vi "运维调试_采配水.vi"() -> ()   [LabVIEW 2016, in "PLC.lvlib"]
uses:
  PLC.lvlib
  <vilib>/Plasmionique/MB Master/MB_Master/MB_Master.lvclass
  <vilib>/Utility/miscctls.llb/LVPointTypeDef.ctl
  <vilib>/Plasmionique/MB Master/MB_Master_Serial/MB_Master_Serial.lvclass
  D:/Program Files (x86)/National Instruments/LabVIEW 2016/vi.lib/Plasmionique/MB Master/MB_Master/MB_Master.lvclass
  <vilib>/Utility/config.llb/Read Key (U32).vi
  <vilib>/Plasmionique/MB Master/MB Master.lvlib
  <vilib>/Utility/config.llb/NI_LVConfig.lvlib
panel:
  out "R21":i16
  in  "V7":bool
  out "R20":i16
  in  "M1-2":bool
  in  "潜水泵工作模式":u16(ring) items=["泵1单泵单管路", "泵2单泵单管路", "双泵双管路"]
  out "X10":bool caption="废液报警"
  out "X9":bool caption="自来水报警"
  out "X8":bool caption="泵2过载报警"
  out "X7":bool caption="泵1过载报警"
  out "X6":bool caption="断电检测"
  out "X5":bool caption="开门检测"
  out "X4":bool caption="烟雾检测"
  out "X3":bool caption="漏水检测"
  out "X2":bool caption="进样检测"
  out "X1":bool
  out "X0":bool caption="采样池液位开关"
  out "Y12":bool caption="多参通电"
  out "R109":i16 caption="配水时间"
  out "集成报警信息":string
  out "R108":i16 caption="自来水报警"
  out "R107":i16 caption="采水池液位报警设置"
  out "R106":i16 caption="进样超时设置"
  out "R105":i16 caption="二级清洗时间"
  out "R104":i16 caption="一级清洗时间"
  out "R103":i16 caption="外部管路清洗时间"
  out "R102":i16 caption="静置沉淀时间"
  out "R101":i16 caption="内部管路润洗时间"
  out "R100":i16 caption="外部管路润洗时间"
  out "R2":i16
  out "R1":i16
  out "多列列表框":i32(listbox)
  out "R19":i16
  in  "V6":bool
  out "R18":i16
  in  "V5":bool
  out "R17":i16
  in  "V4":bool
  out "R16":i16
  in  "V3":bool
  out "R15":i16
  in  "V2":bool
  out "R14":i16
  in  "M2":bool
  out "R13":i16
  in  "V1":bool
  out "R12":i16
  in  "M1-1":bool
  in  "返回":bool
  in  "参数设置":bool
  in  "单步启动":bool
  in  "启动":bool
  in  "停止":bool
  # "S"
  # "S"
  # "S"
  # "S"
  # "S"
  # "S"
  # "S"
  # "S"
  # "S"
  # "S"
  # "单步计时："
  # "s"
  # "流程计时："
  # "s"
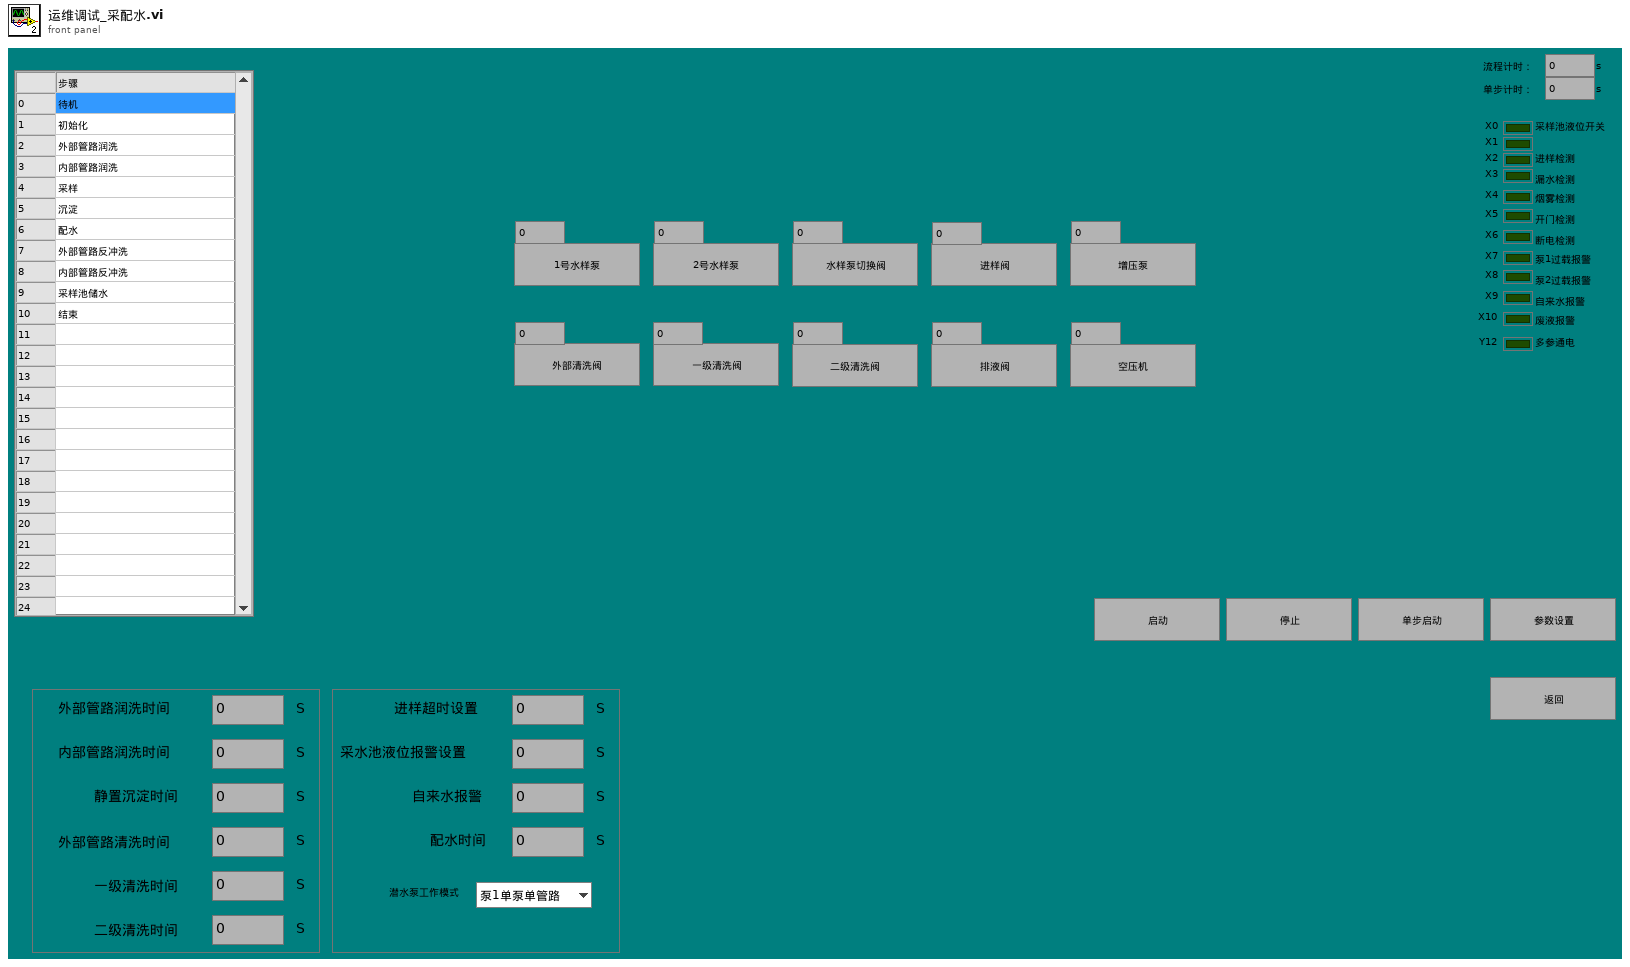
[diagram p1: front panel]
types:
  T1 = typedef "LVPointTypeDef.ctl" = cluster{"Horizontal":i16, "Vertical":i16}
  T2 = cluster{"时间标识":timestamp, "设备":string, "日志信息":string}
  T3 = cluster{"R0":i16, "R1":i16, "R2":i16, "R3":i16, "R4":i16, "R5":i16, "R6":i16, "R7":i16, "R8":i16, "R9":i16, "R10":i16, "R11":i16, "R12":i16, "R13":i16, "R14":i16, "R15":i16, "R16":i16, "R17":i16, "R18":i16, "R19":i16, "R20":i16, "R21":i16}
  T4 = cluster{"coil values[0]":bool, "coil values[1]":bool, "coil values[2]":bool, "coil values[3]":bool, "coil values[4]":bool, "coil values[5]":bool, "coil values[6]":bool, "coil values[7]":bool, "coil values[8]":bool, "coil values[9]":bool, "coil values[10]":bool, "coil values[11]":bool, "coil values[12]":bool, "coil values[13]":bool, "coil values[14]":bool, "coil values[15]":bool}
  T5 = cluster{"seconds since 1Jan1904":timestamp, "table输入":string, string, "table输入":string}
  T6 = cluster{"时间标识":timestamp, "设备":string, "日志信息":string, "流程参数":string}
  T7 = cluster{"命令":string, cluster{"starting address":u16, "holding register value":u16}}
  T8 = cluster{"是否启用仪器":bool, "CODMn":cluster{"启动测量模式":cluster{"测量模式":enum16{"水样测量", "标样核查", "零点核查", "加标回收", "平行样", "校零", "校标"}}, "确定按钮":bool}, "采水模式":enum16{"使用采水泵", "不使用采水泵"}}
  T9 = enum16{"水样测量", "标样核查", "零点核查", "加标回收", "平行样", "校零", "校标"}
  T10 = cluster{"命令":string, "数据":cluster{"starting address":u16, "holding register value":u16}}
  T11 = cluster{"命令":string, "数据":cluster{"starting address":u16, "holding register values":u16[]}}
  T12 = cluster{"命令":string, "data":cluster{"starting address":u16, "coil values":bool[]}}
  T13 = enum32{"Bad", "Idle", "Run top level", "Running"}
  T14 = typedef "NI_LVConfig.lvlib/Config Data RefNum.ctl" = refnum<k1>
  T15 = cluster{"baud rate (bps)":u32, "stop bits":u16, "parity":u16, "flow control":u16, "timeout":u32, "retries":i32}
  T16 = cluster{"starting address":u16, "holding register values":u16[]}
  T17 = cluster{"starting address":u16, "holding register value":u16}
  T18 = cluster{"starting address":u16, "coil values":bool[]}
  T19 = cluster{"Registers[0]":u16, "Registers[1]":u16, "Registers[2]":u16, "Registers[3]":u16, "Registers[4]":u16, "Registers[5]":u16, "Registers[6]":u16, "Registers[7]":u16, "Registers[8]":u16, "Registers[9]":u16, "Registers[10]":u16, "Registers[11]":u16, "Registers[12]":u16, "Registers[13]":u16, "Registers[14]":u16, "Registers[15]":u16, "Registers[16]":u16, "Registers[17]":u16, "Registers[18]":u16, "Registers[19]":u16, "Registers[20]":u16, "Registers[21]":u16}
  T20 = cluster{"Registers[0]":u16, "Registers[1]":u16, "Registers[2]":u16, "Registers[3]":u16, "Registers[4]":u16, "Registers[5]":u16}
  T21 = cluster{"Coils[0]":bool, "Coils[1]":bool, "Coils[2]":bool, "Coils[3]":bool, "Coils[4]":bool, "Coils[5]":bool, "Coils[6]":bool, "Coils[7]":bool, "Coils[8]":bool, "Coils[9]":bool, "Coils[10]":bool, "Coils[11]":bool, "Coils[12]":bool, "Coils[13]":bool, "Coils[14]":bool, "Coils[15]":bool}
  T22 = cluster{"Registers[0]":u16, "Registers[1]":u16, "Registers[2]":u16, "Registers[3]":u16, "Registers[4]":u16, "Registers[5]":u16, "Registers[6]":u16, "Registers[7]":u16, "Registers[8]":u16, "Registers[9]":u16, "Registers[10]":u16, "Registers[11]":u16, "Registers[12]":u16, "Registers[13]":u16, "Registers[14]":u16, "Registers[15]":u16, "Registers[16]":u16, "Registers[17]":u16, "Registers[18]":u16, "Registers[19]":u16}
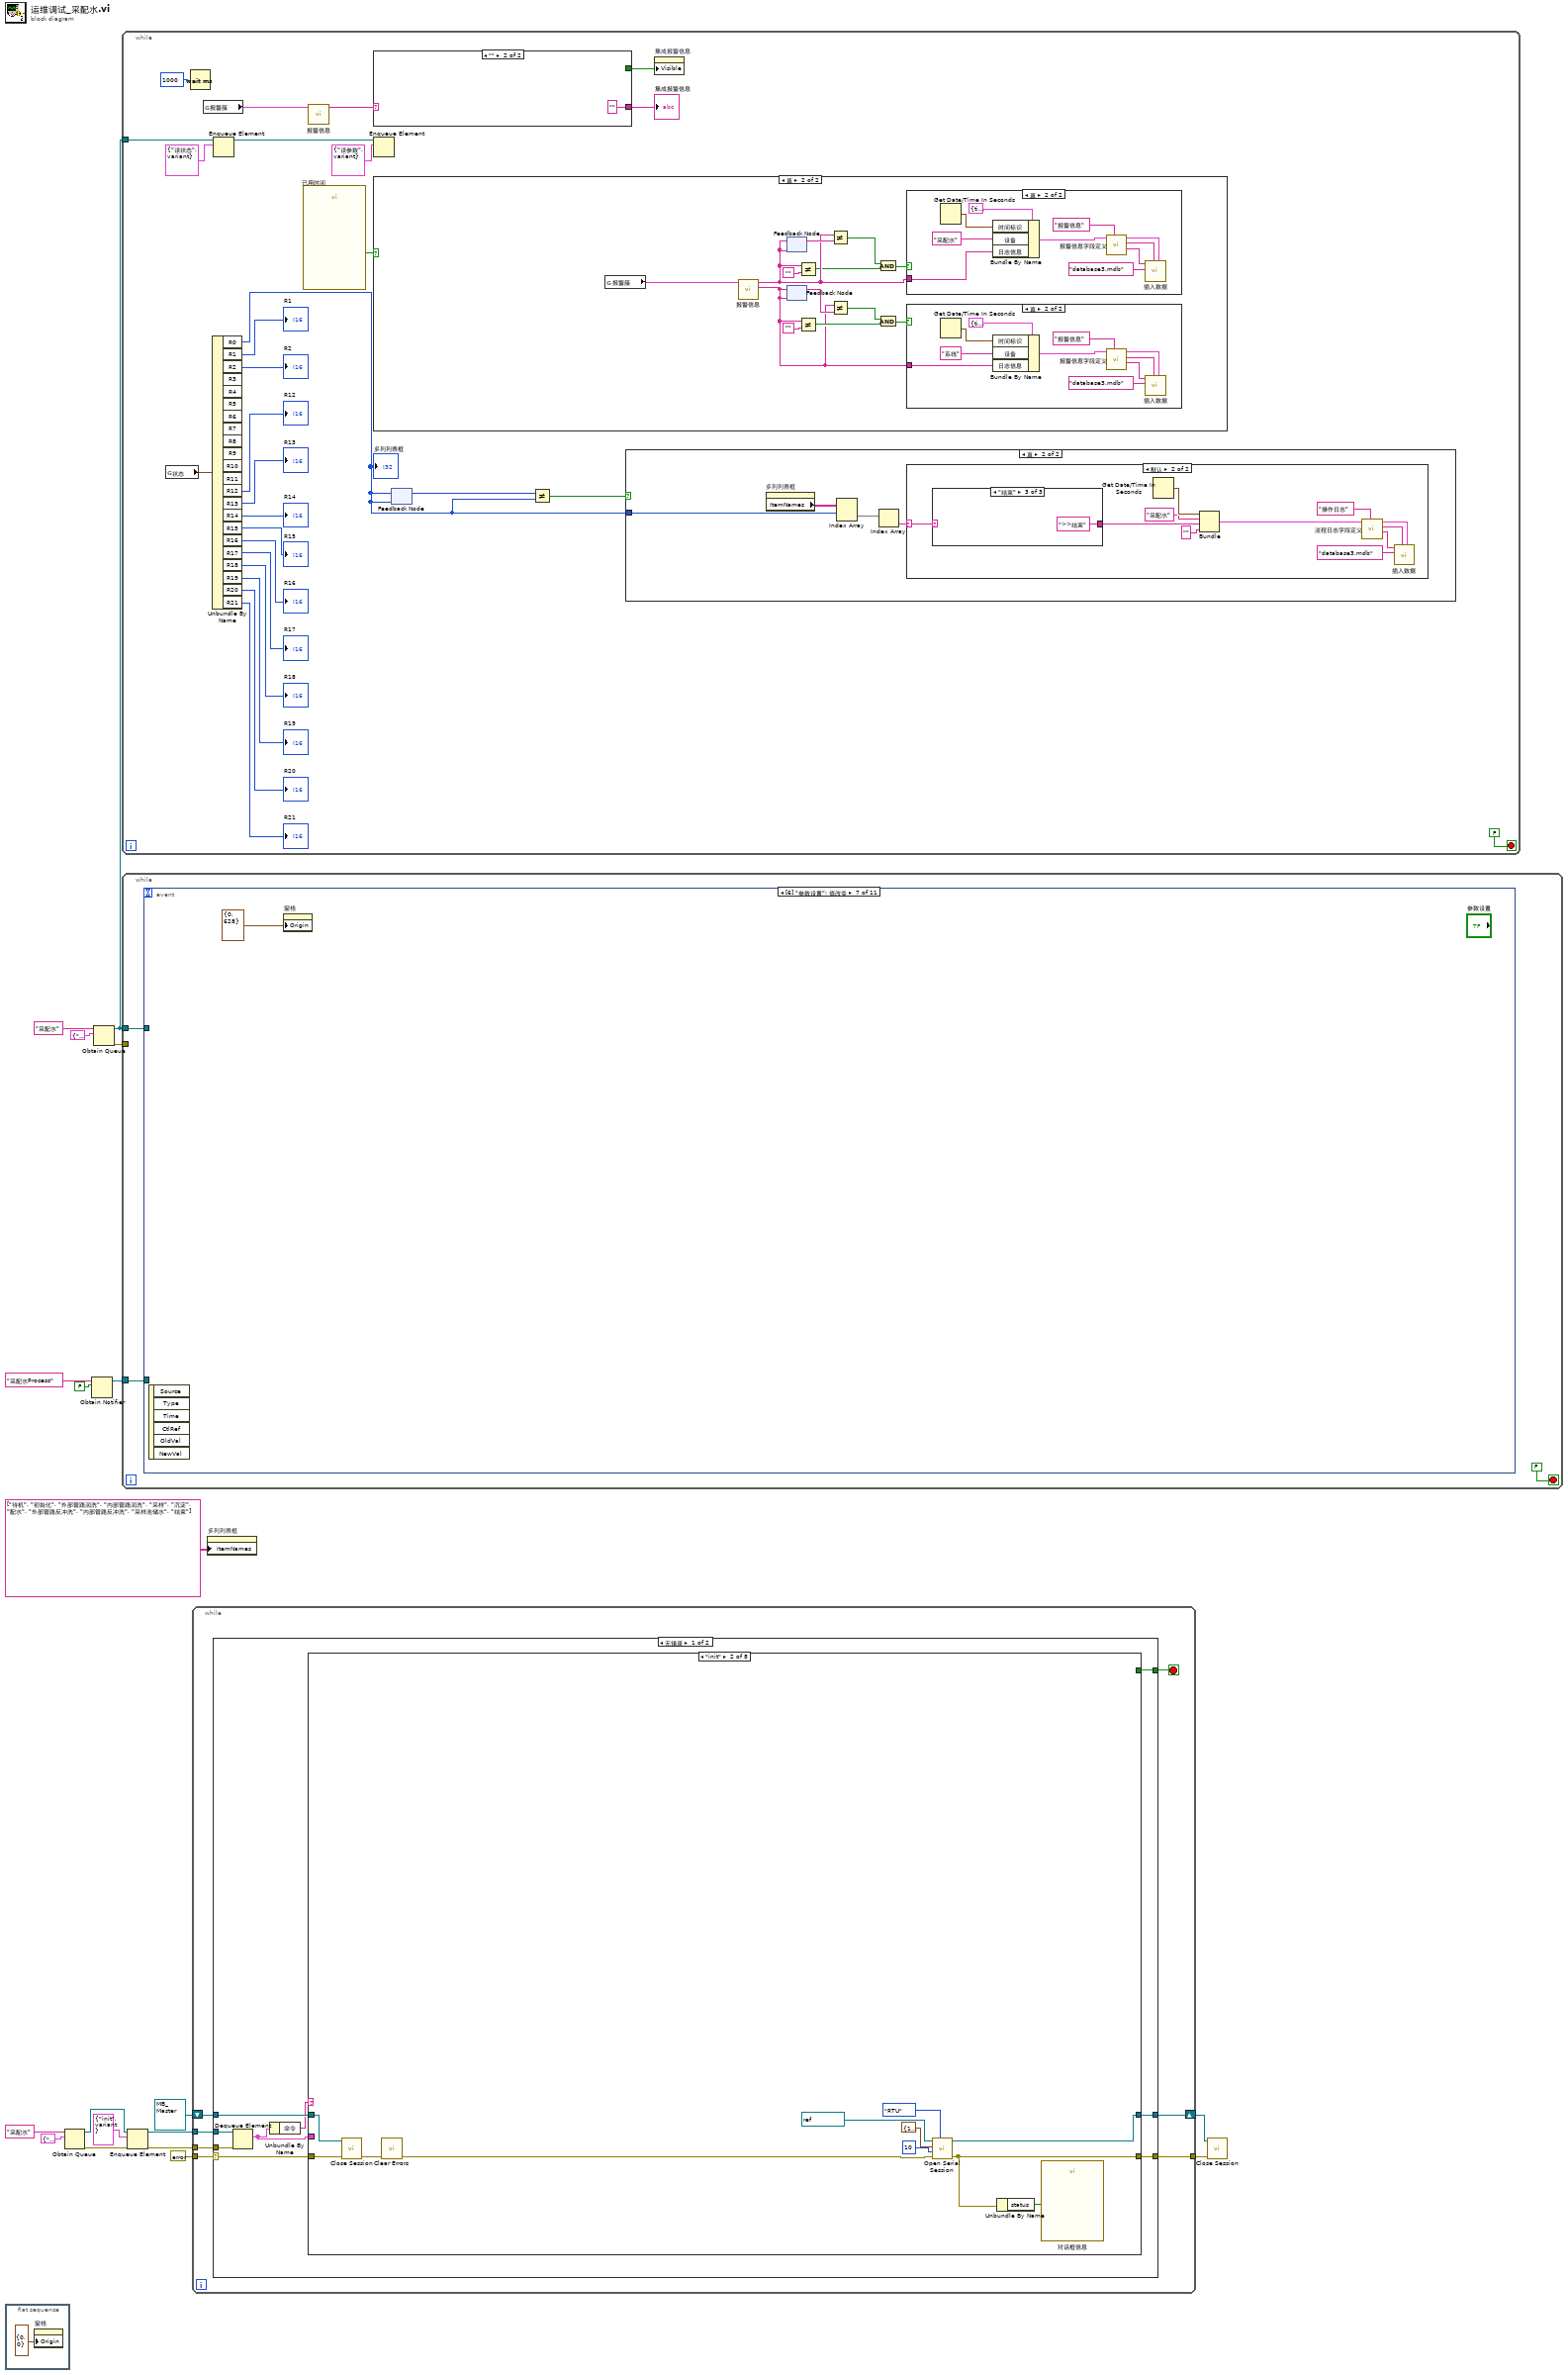
[diagram p0: block diagram]
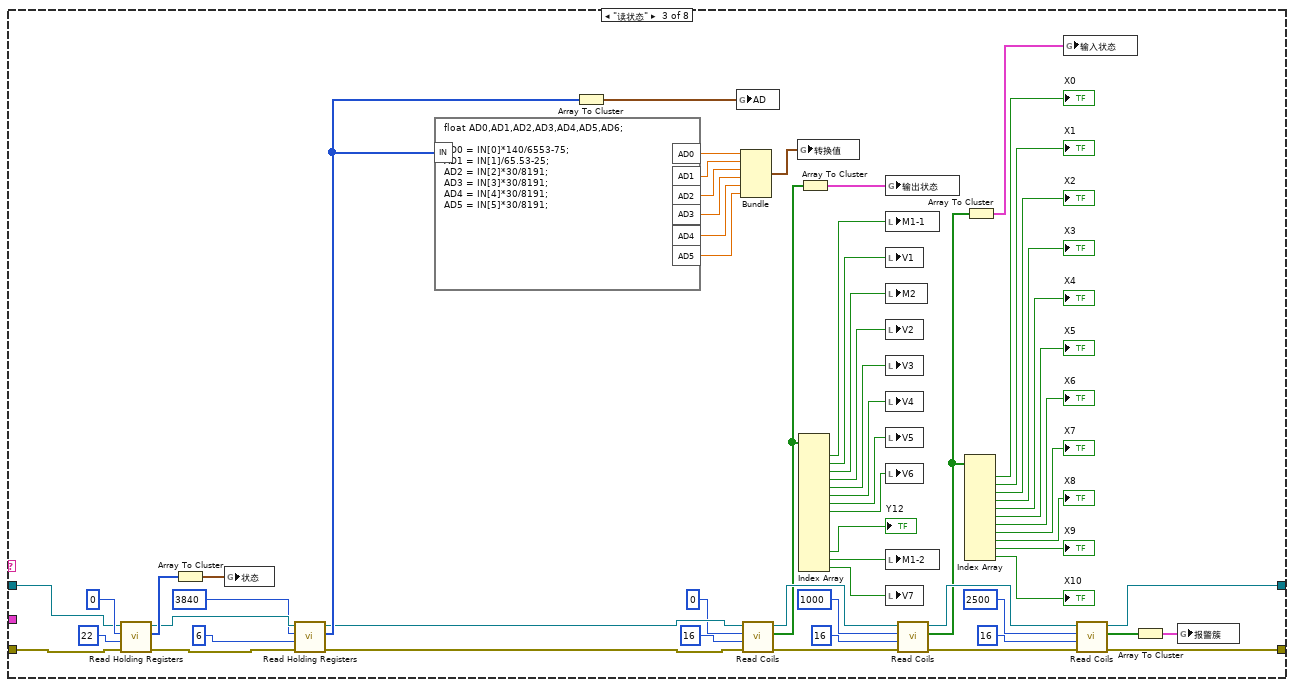
[diagram p3: hidden frame]
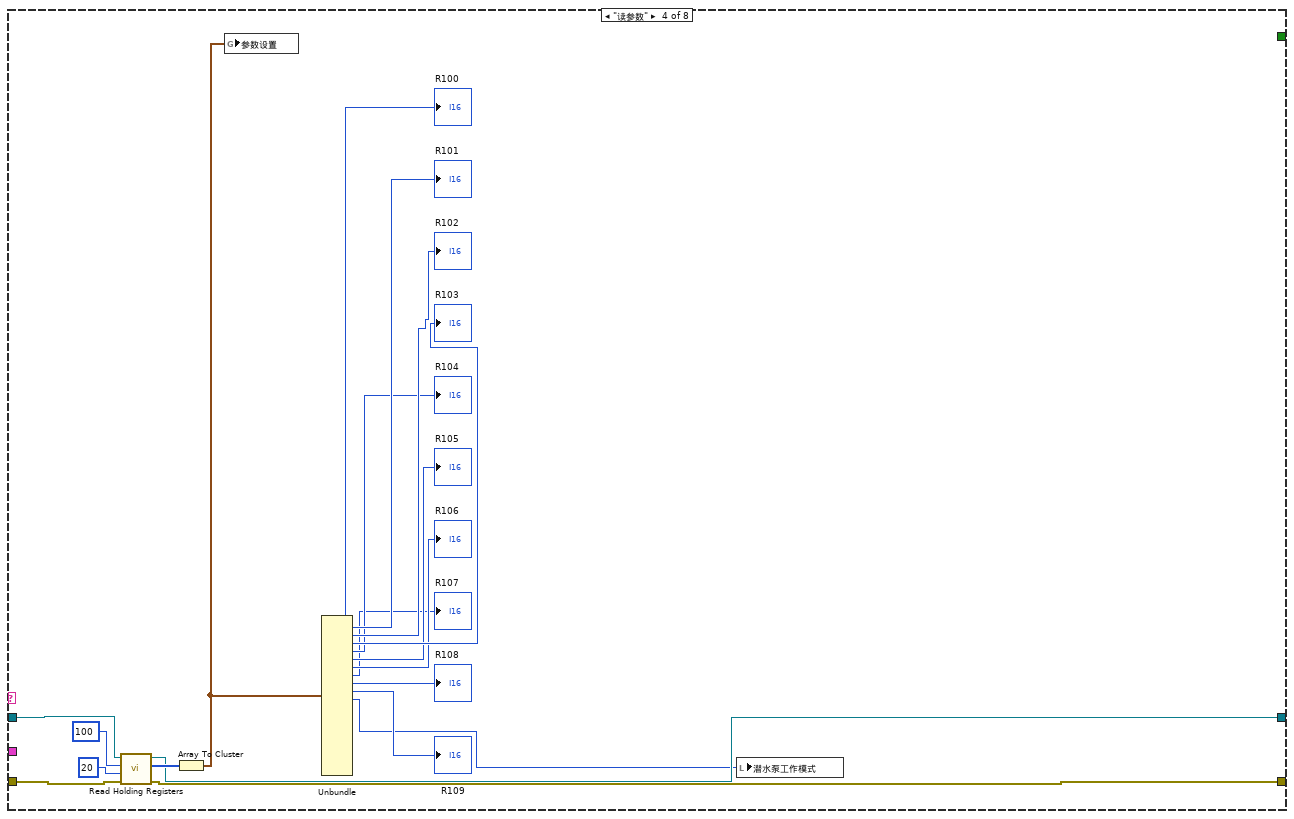
[diagram p4: hidden frame]
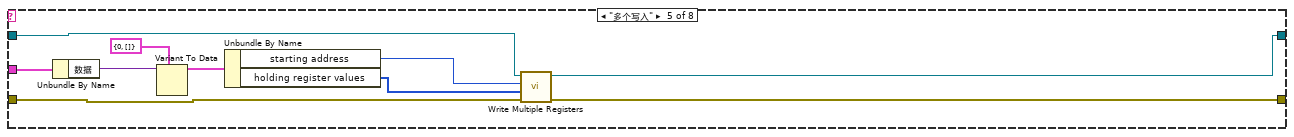
[diagram p5: hidden frame]
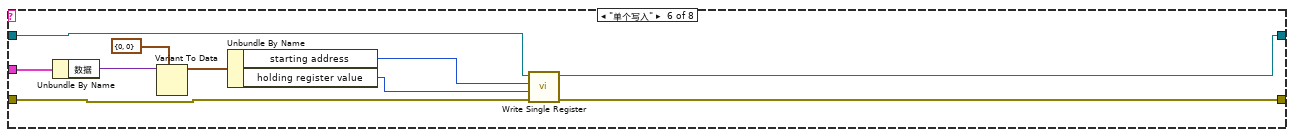
[diagram p6: hidden frame]
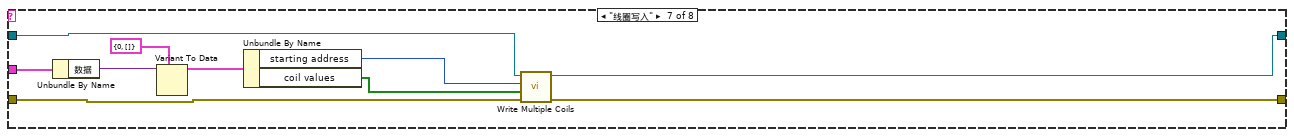
[diagram p7: hidden frame]
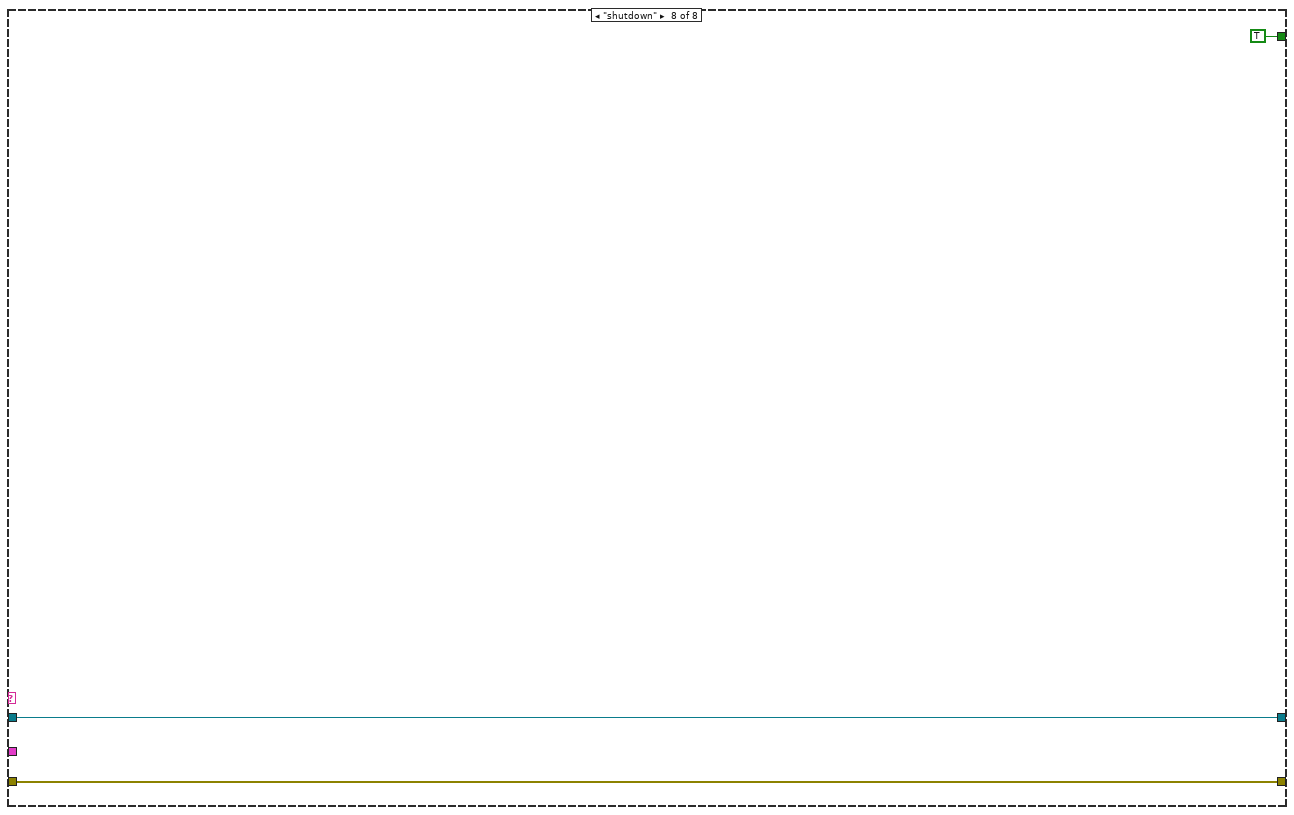
[diagram p8: hidden frame]
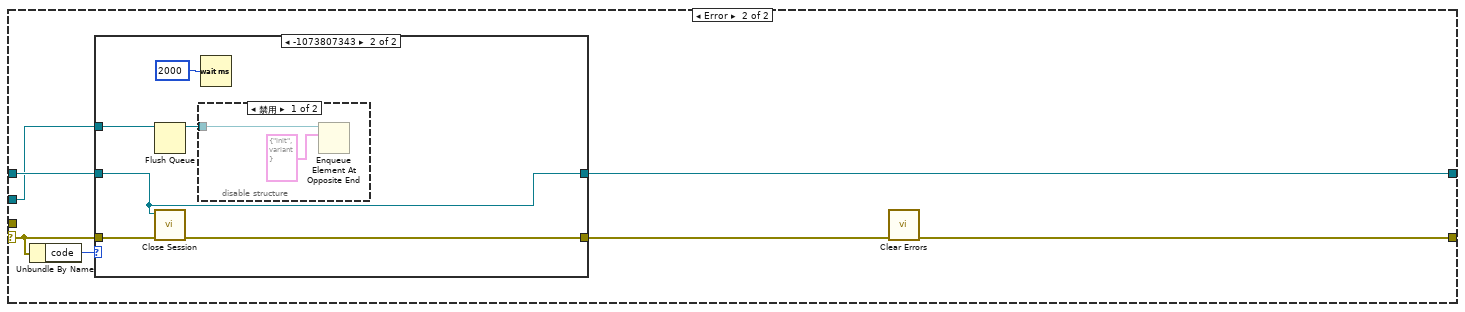
[diagram p9: hidden frame]
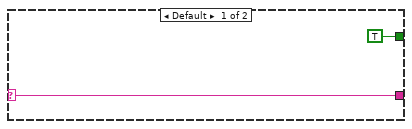
[diagram p15: hidden frame]
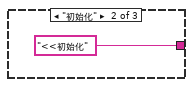
[diagram p19: hidden frame]
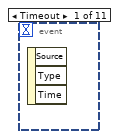
[diagram p20: hidden frame]
diagram:
  n1 = flat-sequence {
    frame #0 {
      n2 = property on="窗格" class="Pane"("Origin"=T1 {"Horizontal"=0, "Vertical"=0} ("原点")) -> ()  [unwired: 2 in, 2 out]
    }
  }
  n3 = Obtain Queue(name (unnamed)="采配水" ("名称（未命名）"), element data type=cluster{"命令":string, "数据":variant} {"命令"="", "数据"=variant}) -> (queue out=w9:refnum<queue>, error out=w8:errorcluster)  [unwired: 3 in, 1 out]
  n4 = Obtain Notifier(name (unnamed)="采配水Process" ("名称（未命名）"), notification data type=FALSE) -> (notifier out=w12:refnum<notifier>)  [unwired: 2 in, 2 out]
  n5 = Obtain Queue(name (unnamed)="采配水" ("名称（未命名）"), element data type=cluster{"命令":string, "数据":variant} {"命令"="", "数据"=variant}) -> (queue out=w16:refnum<queue>, error out=w17:errorcluster)  [unwired: 3 in, 1 out]
  n6 = while {
    tunnel: w16 -> [w46]
    stop <- FALSE stop-if-true
    n7 = global read "采配水全局变量.vi" "状态"() -> (w44:T3)
    n8 = Wait (ms)(milliseconds to wait=u32 1000 ("等待时间（毫秒）")) -> ()  [unwired: 1 out]
    n9 = global read "采配水全局变量.vi" "报警簇"() -> (w32:T4)
    n10 = Unbundle By Name(w44) -> ("R0"=w24:i16, "R1"=→"R1":i16, "R2"=→"R2":i16, "R12"=→"R12":i16, "R13"=→"R13":i16, "R14"=→"R14":i16, "R15"=→"R15":i16, "R16"=→"R16":i16, "R17"=→"R17":i16, "R18"=→"R18":i16, "R19"=→"R19":i16, "R20"=→"R20":i16, "R21"=→"R21":i16)  [unwired: 9 out]
    "多列列表框" <- w24
    n11 = Enqueue Element(queue=w46, element=cluster{"命令":string, "数据":variant} {"命令"="读状态", "数据"=variant} ("元素")) -> (queue out=w26:refnum<queue>)  [unwired: 2 in, 2 out]
    n12 = call "已用时间"() -> ("Time has Elapsed"=w29:bool)  [unwired: 12 in, 7 out]
    n13 = call "报警信息.vi"("报警簇"=w32) -> ("采配水报警信息"=w23:string)  [unwired: 9 in, 1 out]
    n14 = case shown="\"\"" w23 {
      selector: w23 -> [w82 _]
      tunnel: [w82 "" ("字符串")] -> w31
      tunnel: [TRUE ("可见") _] -> w30
      frame Default {
      }
      frame "" {
      }
    }
    "集成报警信息" <- w31
    n15 = Enqueue Element(queue=w26, element=cluster{"命令":string, "数据":variant} {"命令"="读参数", "数据"=variant} ("元素")) -> ()  [unwired: 2 in, 3 out]
    n16 = case shown="真" w29 {
      frame False {
      }
      frame True {
        n17 = global read "采配水全局变量.vi" "报警簇"() -> (w60:T4)
        n18 = call "报警信息.vi"("报警簇"=w60) -> ("系统报警信息"=w49:string, "采配水报警信息"=w56:string)  [unwired: 9 in]
        n19 = feedback #1(w56) -> (w59:string)
        n20 = feedback-in #1(w56) -> ()
        n21 = feedback #2(w49) -> (w50:string)
        n22 = feedback-in #2(w49) -> ()
        n23 = Not Equal?(x=w56, y="") -> (x != y?=w54:bool)
        n24 = Not Equal?(x=w49, y="") -> (x != y?=w53:bool)
        n25 = Not Equal?(x=w56, y=w59) -> (x != y?=w58:bool)
        n26 = Not Equal?(x=w49, y=w50) -> (x != y?=w51:bool)
        n27 = And(x=w58, y=w54) -> (x .and. y?=w57:bool)
        n28 = And(x=w51, y=w53) -> (x .and. y?=w48:bool)
        n29 = case shown="真" w57 {
          tunnel: w56 -> [_ w71]
          frame False {
          }
          frame True {
            n30 = Get Date/Time In Seconds() -> (seconds since 1Jan1904=w73:timestamp)
            n31 = Bundle By Name(cluster=T2 {"时间标识"=timestamp(0 s since 1904-01-01), "设备"="", "日志信息"=""} ("data in"), "时间标识"=w73, "设备"="采配水", "日志信息"=w71) -> (w74:T2)
            n32 = call "报警信息字段定义.vi"("table输入"="报警信息", "data in"=w74) -> ("table输出"=w78:string, "columns"=w79:string[], "data out"=w80:T2)  [unwired: 7 in]
            n33 = call "插入数据.vi"("data"=w80, "columns"=w79, "database"="database3.mdb", "table"=w78) -> ()  [unwired: 7 in, 1 out]
          }
        }
        n34 = case shown="真" w48 {
          tunnel: w49 -> [_ w61]
          frame False {
          }
          frame True {
            n35 = Get Date/Time In Seconds() -> (seconds since 1Jan1904=w63:timestamp)
            n36 = Bundle By Name(cluster=T2 {"时间标识"=timestamp(0 s since 1904-01-01), "设备"="", "日志信息"=""} ("data in"), "时间标识"=w63, "设备"="系统", "日志信息"=w61) -> (w64:T2)
            n37 = call "报警信息字段定义.vi"("table输入"="报警信息", "data in"=w64) -> ("table输出"=w68:string, "columns"=w69:string[], "data out"=w70:T2)  [unwired: 7 in]
            n38 = call "插入数据.vi"("data"=w70, "columns"=w69, "database"="database3.mdb", "table"=w68) -> ()  [unwired: 7 in, 1 out]
          }
        }
      }
    }
    n39 = feedback-in #3(w24) -> ()
    n40 = feedback #3(w24) -> (w25:i16)
    n41 = Not Equal?(x=w25, y=w24) -> (x != y?=w33:bool)
    n42 = case shown="真" w33 {
      tunnel: w24 -> [_ w86]
      frame False {
      }
      frame True {
        n43 = property on="多列列表框" class="MCListbox (严格)"() -> ("ItemNames"=w87:string[][])  [unwired: 2 in, 2 out]
        n44 = Index Array(array=w87, index (row)=w86) -> (element=w85:string[])  [unwired: 1 in]
        n45 = Index Array(array=w85) -> (element=w84:string)  [unwired: 1 in]
        n46 = case shown="默认" w84 {
          selector: w84 -> [_ w89]
          frame "待机" {
          }
          frame Default {
            n47 = case shown="\"结束\"" w89 {
              selector: w89 -> [w99 _ _]
              tunnel: [w99 "<<初始化" ">>结束"] -> w88
              frame Default {
              }
              frame "初始化" {
              }
              frame "结束" {
              }
            }
            n48 = Get Date/Time In Seconds() -> (seconds since 1Jan1904=w93:timestamp)
            n49 = Bundle("seconds since 1Jan1904"=w93, "table输入"="采配水", w88, "table输入"="") -> (w91:T5)  [unwired: 1 in]
            n50 = call "流程日志字段定义.vi"("table输入"="操作日志", "data in"=w91) -> ("table输出"=w96:string, "columns"=w97:string[], "data out"=w98:T6)  [unwired: 7 in]
            n51 = call "插入数据.vi"("data"=w98, "columns"=w97, "database"="database3.mdb", "table"=w96) -> ()  [unwired: 7 in, 1 out]
          }
        }
      }
    }
    n52 = property on="集成报警信息" class="Str"("Visible"=w30) -> ()  [unwired: 2 in, 2 out]
  }
  n53 = while {
    tunnel: w16 -> [w103]
    tunnel: w17 -> [_]
    tunnel: w12 -> [w102]
    stop <- FALSE stop-if-true
    n54 = event shown="[6] \"参数设置\": 值改变" {
      selector: _ -> [_ _ _ _ _ _ _ _ _ _ _]
      dyn-events: _ -> [_ _ _ _ _ _ _ _ _ _ _]
      timeout: _ -> [_ _ _ _ _ _ _ _ _ _ _]
      tunnel: w103 -> [_ w107 w110 w145 w161 _ _ _ w179 w181 w186]
      tunnel: w102 -> [_ w106 w109 _ _ _ _ _ _ _ _]
      event Timeout {
        n55 = event-data() -> ()  [unwired: 1 in, 3 out]
      }
      event "停止": Value Change {
        n56 = event-data() -> ()  [unwired: 1 in, 6 out]
        n57 = Send Notification(notification=TRUE ("通知"), notifier=w106) -> ()  [unwired: 1 in, 2 out]
        n58 = Enqueue Element At Opposite End(queue=w107, element=T7 {"命令"="单个写入", {"starting address"=300, "holding register value"=2}} ("元素")) -> ()  [unwired: 2 in, 3 out]
      }
      event "启动": Value Change {
        n59 = event-data() -> ()  [unwired: 1 in, 6 out]
        n60 = disable-structure shown="禁用" {
          disable-tunnel: w110 -> [w141 _]
          frame Disabled {
            n61 = Enqueue Element At Opposite End(queue=w141, element=T7 {"命令"="单个写入", {"starting address"=300, "holding register value"=1}} ("元素")) -> ()  [unwired: 2 in, 3 out]
          }
          frame Enabled {
          }
        }
        n62 = flat-sequence {
          tunnel: w109 -> [w111]
          frame #0 {
            n63 = Cancel Notification(0:w111) -> ()  [unwired: 1 in, 3 out]
          }
          frame #1 {
            n64 = vi-ref "一体站流程自动启动.vi"() -> (w114:refnum<vi>)
            n65 = property class="VI"(reference=w114) -> ("Name"=w113:string, "Exec.State"=w112:T13)  [unwired: 1 in, 2 out]
            n66 = case shown="\"Idle\"" w112 {
              tunnel: w113 -> [_ w138 _ _]
              frame "Bad", Default {
              }
              frame "Idle" {
                n67 = call <vilib>:"Application Directory.vi"() -> ("Application Directory"=w122:path)
                n68 = Build Path(base path=w122, name or relative path="data\\Set.ini" ("名称或相对路径")) -> (appended path=w120:path)
                n69 = call <vilib>:"Open Config Data.vi"("configuration file path"=w120) -> ("error out"=w123:errorcluster, "refnum"=w124:T14)  [unwired: 8 in, 1 out]
                n70 = call-poly <vilib>:"Read Key.vi"("section"="系统设置", "error in (no error)"=w123, "key"="采水模式", "refnum"=w124) -> ("error out"=w118:errorcluster, "value"=w115:u32, "refnum out"=w119:T14)  [unwired: 4 in, 1 out]
                n71 = call <vilib>:"Close Config Data.vi"("error in (no error)"=w118, "refnum"=w119) -> ()  [unwired: 8 in, 2 out]
                n72 = Two Button Dialog(message="请选择是否启用仪器测量" ("消息"), 1:"不启用" ("F按钮名称（“取消”）"), 2:"启用" ("T按钮名称（“确定”）")) -> (T button?=w128:bool)
                n73 = Bundle By Name(cluster=T8 {"是否启用仪器"=FALSE, "CODMn"={"启动测量模式"={"测量模式"=enum."水样测量"}, "确定按钮"=FALSE}, "采水模式"=enum."使用采水泵"} ("参数"), "是否启用仪器"=w128, "CODMn.启动测量模式.测量模式"=T9."水样测量", "采水模式"=w115) -> (w125:T8)
                n74 = Open VI Reference(type specifier VI Refnum (for type only)=refnum<vi> refnum, vi path=w138, options=128 ("选项")) -> (vi reference=w136:refnum<vi>, error out=w133:errorcluster)  [unwired: 3 in]
                n75 = call-by-ref "开始异步调用"(reference=w136, error in=w133, "参数"=w125) -> (reference out=w134:refnum<vi>, error out=w132:errorcluster)  [unwired: 11 in]
                n76 = Close Reference(reference=w134, error in (no error)=w132) -> ()  [unwired: 1 out]
              }
              frame "Run top level" {
              }
              frame "Running" {
                n77 = One Button Dialog(message="流程已经运行,无须重复启动" ("消息")) -> ()  [unwired: 1 in, 1 out]
              }
            }
          }
        }
      }
      event "单步启动": Value Change {
        n78 = event-data() -> ()  [unwired: 1 in, 6 out]
        n79 = call "单步启动对话框.vi"() -> ("单步启动步骤输出"=w142:u16)  [unwired: 11 in]
        n80 = Bundle By Name(cluster=T10 {"命令"="单个写入", "数据"={"starting address"=301, "holding register value"=0}} ("元素"), "数据.holding register value"=w142) -> (w143:T10)
        n81 = Enqueue Element At Opposite End(queue=w145, element=w143) -> ()  [unwired: 2 in, 3 out]
      }
      event "R100", "R101", "R102", "R103", "R104", "R105", "R106", "R107", "R108", "R109", "潜水泵工作模式": Value Change {
        n82 = event-data() -> ()  [unwired: 1 in, 6 out]
        n83 = local read "R100"() -> (w156:i16)
        n84 = local read "R101"() -> (w155:i16)
        n85 = local read "R102"() -> (w154:i16)
        n86 = local read "R103"() -> (w153:i16)
        n87 = local read "R104"() -> (w152:i16)
        n88 = local read "R105"() -> (w151:i16)
        n89 = local read "R106"() -> (w150:i16)
        n90 = local read "R107"() -> (w149:i16)
        n91 = local read "R108"() -> (w148:i16)
        n92 = local read "R109"() -> (w147:i16)
        n93 = Build Array(w156, w155, w154, w153, w152, w151, w150, w149, w148, w147, "潜水泵工作模式") -> (w157:u16[])
        n94 = Bundle By Name(cluster=T11 {"命令"="多个写入", "数据"={"starting address"=0, "holding register values"=[]}} ("元素"), "数据.starting address"=u16 100, "数据.holding register values"=w157) -> (w158:T11)
        n95 = Enqueue Element At Opposite End(queue=w161, element=w158) -> ()  [unwired: 2 in, 3 out]
      }
      event "R100", "R101", "R102", "R103", "R104", "R105", "R106", "R107", "R108", "R109": Mouse Down {
        n96 = event-data() -> ("CtlRef"=w165:refnum<vi>)  [unwired: 1 in, 7 out]
        n97 = property class="DigNum (严格)"(reference=w165) -> (reference out=w163:refnum<vi>, "Value"=w164:i16)  [unwired: 1 in, 1 out]
        n98 = call "数字键盘.vi"("OldNumber"=w164) -> ("NewNumber"=w162:sgl)
        n99 = property class="DigNum (严格)"(reference=w163, "Val(Sgnl)"=w162) -> ()  [unwired: 1 in, 2 out]
      }
      event "参数设置": Value Change {
        n100 = event-data() -> ()  [unwired: 1 in, 6 out]
        n101 = property on="窗格" class="Pane"("Origin"=T1 {"Horizontal"=0, "Vertical"=628} ("原点")) -> ()  [unwired: 2 in, 2 out]
      }
      event "返回": Value Change {
        n102 = event-data() -> ()  [unwired: 1 in, 6 out]
        n103 = property on="窗格" class="Pane"("Origin"=T1 {"Horizontal"=0, "Vertical"=0} ("原点")) -> ()  [unwired: 2 in, 2 out]
      }
      event "M1-1", "V1", "M2", "V2", "V3", "V4", "V5", "V6": Value Change {
        n104 = event-data() -> ()  [unwired: 1 in, 6 out]
        n105 = Build Array("M1-1", "V1", "M2", "V2", "V3", "V4", "V5", "V6") -> (w168:bool[])
        n106 = Bundle By Name(cluster=T12 {"命令"="线圈写入", "data"={"starting address"=2400, "coil values"=[]}} ("元素"), "data.coil values"=w168) -> (w169:T12)
        n107 = Enqueue Element(queue=w179, element=w169) -> ()  [unwired: 2 in, 3 out]
      }
      event "M1-2": Value Change {
        n108 = event-data() -> ()  [unwired: 1 in, 6 out]
        n109 = Build Array("M1-2") -> (w182:bool[])
        n110 = Bundle By Name(cluster=T12 {"命令"="线圈写入", "data"={"starting address"=2413, "coil values"=[]}} ("元素"), "data.coil values"=w182) -> (w183:T12)
        n111 = Enqueue Element(queue=w181, element=w183) -> ()  [unwired: 2 in, 3 out]
      }
      event "V7": Value Change {
        n112 = event-data() -> ()  [unwired: 1 in, 6 out]
        n113 = Build Array("V7") -> (w187:bool[])
        n114 = Bundle By Name(cluster=T12 {"命令"="线圈写入", "data"={"starting address"=2413, "coil values"=[]}} ("元素"), "data.coil values"=w187) -> (w188:T12)
        n115 = Enqueue Element(queue=w186, element=w188) -> ()  [unwired: 2 in, 3 out]
      }
    }
  }
  n116 = Enqueue Element(queue=w9, element=cluster{"命令":string, "数据":variant} {"命令"="init", "数据"=variant} ("元素"), error in (no error)=w8) -> (queue out=w4:refnum<queue>, error out=w6:errorcluster)  [unwired: 1 in, 1 out]
  n117 = while {
    tunnel: w4 -> [w192]
    tunnel: w6 -> [w191]
    shift-right: [w196] -> w1
    shift-left: refnum<class "MB_Master.lvclass"> refnum ("MB session in") -> [w195]
    tunnel: errorcluster {"status"=FALSE, "code"=0, "source"=""} ("error out") -> [w193]
    tunnel: [w194] -> w2
    stop <- w190 stop-if-true
    n118 = case shown="无错误" w193 {
      selector: w193 -> [w202 w336]
      tunnel: [w205 w335] -> w196
      tunnel: w195 -> [w204 w337]
      tunnel: [w203 w333] -> w194
      tunnel: w192 -> [w199 w332]
      tunnel: w191 -> [w198 _]
      tunnel: [w200 _] -> w190
      frame No Error {
        n119 = Dequeue Element(queue=w199, error in (no error)=w198) -> (element=w197:cluster{"命令":string, "数据":variant})  [unwired: 1 in, 3 out]
        n120 = Unbundle By Name(w197) -> ("命令"=w201:string)
        n121 = case shown="\"init\"" w201 {
          tunnel: [w207 w211 w244 w293 w305 w315 w325 w330] -> w205
          tunnel: w204 -> [w207 w215 w264 w298 w308 w318 w328 w330]
          tunnel: [w206 w213 w243 w292 w306 w316 w326 w329] -> w203
          tunnel: w202 -> [w206 w217 w267 w297 w307 w317 w327 w329]
          tunnel: [_ _ _ _ _ _ _ TRUE] -> w200
          tunnel: w197 -> [_ _ _ _ w304 w314 w324 _]
          frame "idle", Default {
          }
          frame "init" {
            n122 = call-dynamic "Close Session.vi"("error in (no error)"=w217, "MB session in"=w215) -> ("error out"=w216:errorcluster)  [unwired: 9 in]
            n123 = call <vilib>:"Clear Errors.vi"("error in (no error)"=w216) -> ("error out"=w214:errorcluster)  [unwired: 5 in, 1 out]
            n124 = call <vilib>:"Open Serial Session.vi"("Mode (RTU)"=enum16{"RTU", "ASCII"}."RTU", "Error in"=w214, "Slave ID"=u8 10, "Serial Config"=T15 {"baud rate (bps)"=115200, "stop bits"=10, "parity"=0, "flow control"=0, "timeout"=100, "retries"=1}, "VISA Resource"=refnum<visa-resource-name> "COM3" ("VISA resource name")) -> ("Error out"=w213:errorcluster, "MB_Serial session"=w211:refnum<class "MB_Master_Serial.lvclass">)  [unwired: 5 in]
            n125 = Unbundle By Name(w213) -> ("status"=w218:bool)
            n126 = call "对话框信息"("Enable"=w218) -> ()  [unwired: 9 in, 2 out]
          }
          frame "读状态" {
            n127 = call <vilib>:"Read Holding Registers.vi"("error in (no error)"=w267, "quantity"=u16 22 ("number of holding registers"), "starting address"=u16 0, "MB session in"=w264) -> ("error out"=w260:errorcluster, "Registers"=w263:u16[], "MB session out"=w262:refnum<class "MB_Master.lvclass">)  [unwired: 5 in]
            n128 = Array To Cluster(array=w263) -> (cluster=w269:T19)
            n129 = global write "采配水全局变量.vi" "状态"(w269) -> ()
            n130 = call <vilib>:"Read Holding Registers.vi"("error in (no error)"=w260, "quantity"=u16 6 ("number of holding registers"), "starting address"=u16 3840, "MB session in"=w262) -> ("error out"=w256:errorcluster, "Registers"=w261:u16[], "MB session out"=w257:refnum<class "MB_Master.lvclass">)  [unwired: 5 in]
            n131 = formula code="float AD0,AD1,AD2,AD3,AD4,AD5,AD6;\n\nAD0 = IN[0]*140/6553-75;\nAD1 = IN[1]/65.53-25;\nAD2 = IN[2]*30/8191;\nAD3 = IN[3]*30/8191;\nAD4 = IN[4]*30/8191;\nAD5 = IN[5]*30/8191;"("IN"=w261) -> ("AD0"=w275:dbl, "AD1"=w274:dbl, "AD2"=w273:dbl, "AD3"=w272:dbl, "AD4"=w271:dbl, "AD5"=w270:dbl)
            n132 = Array To Cluster(array=w261) -> (cluster=w277:T20)
            n133 = global write "采配水全局变量.vi" "AD"(w277) -> ()
            n134 = Bundle(w275, w274, w273, w272, w271, w270) -> (w276:cluster{dbl, dbl, dbl, dbl, dbl, dbl})  [unwired: 1 in]
            n135 = call <vilib>:"Read Coils.vi"("error in (no error)"=w256, "quantity"=u16 16 ("number of coils"), "starting address"=u16 0, "MB session in"=w257) -> ("error out"=w252:errorcluster, "Coils"=w233:bool[], "MB session out"=w253:refnum<class "MB_Master.lvclass">)  [unwired: 5 in]
            n136 = global write "采配水全局变量.vi" "转换值"(w276) -> ()
            n137 = Index Array(array=w233) -> (element #1=w228:bool, element #2=w227:bool, element #3=w226:bool, element #4=w225:bool, element #5=w224:bool, element #6=w223:bool, element #7=w222:bool, element #8=w221:bool, element #13=→"Y12":bool, element #14=w220:bool, element #15=w219:bool)  [unwired: 15 in, 4 out]
            n138 = Array To Cluster(array=w233) -> (cluster=w278:T21)
            n139 = global write "采配水全局变量.vi" "输出状态"(w278) -> ()
            n140 = local write "M1-1"(w228) -> ()
            n141 = local write "V1"(w227) -> ()
            n142 = local write "M2"(w226) -> ()
            n143 = local write "V2"(w225) -> ()
            n144 = local write "V3"(w224) -> ()
            n145 = local write "V4"(w223) -> ()
            n146 = local write "V5"(w222) -> ()
            n147 = local write "V6"(w221) -> ()
            n148 = local write "M1-2"(w220) -> ()
            n149 = local write "V7"(w219) -> ()
            n150 = call <vilib>:"Read Coils.vi"("error in (no error)"=w252, "quantity"=u16 16 ("number of coils"), "starting address"=u16 1000, "MB session in"=w253) -> ("error out"=w248:errorcluster, "Coils"=w242:bool[], "MB session out"=w249:refnum<class "MB_Master.lvclass">)  [unwired: 5 in]
            n151 = Index Array(array=w242) -> (element #1=→"X0":bool, element #2=→"X1":bool, element #3=→"X2":bool, element #4=→"X3":bool, element #5=→"X4":bool, element #6=→"X5":bool, element #7=→"X6":bool, element #8=→"X7":bool, element #9=→"X8":bool, element #10=→"X9":bool, element #11=→"X10":bool)  [unwired: 11 in]
            n152 = Array To Cluster(array=w242) -> (cluster=w279:T21)
            n153 = global write "采配水全局变量.vi" "输入状态"(w279) -> ()
            n154 = call <vilib>:"Read Coils.vi"("error in (no error)"=w248, "quantity"=u16 16 ("number of coils"), "starting address"=u16 2500, "MB session in"=w249) -> ("error out"=w243:errorcluster, "Coils"=w245:bool[], "MB session out"=w244:refnum<class "MB_Master.lvclass">)  [unwired: 5 in]
            n155 = Array To Cluster(array=w245) -> (cluster=w268:T21)
            n156 = global write "采配水全局变量.vi" "报警簇"(w268) -> ()
          }
          frame "读参数" {
            n157 = call <vilib>:"Read Holding Registers.vi"("error in (no error)"=w297, "quantity"=u16 20 ("number of holding registers"), "starting address"=u16 100, "MB session in"=w298) -> ("error out"=w292:errorcluster, "Registers"=w294:u16[], "MB session out"=w293:refnum<class "MB_Master.lvclass">)  [unwired: 5 in]
            n158 = Array To Cluster(array=w294) -> (cluster=w281:T22)
            n159 = global write "采配水全局变量.vi" "参数设置"(w281) -> ()
            n160 = Unbundle(w281) -> ("Registers[0]"=→"R100":u16, "Registers[1]"=→"R101":u16, "Registers[2]"=→"R102":u16, "Registers[3]"=→"R103":u16, "Registers[4]"=→"R104":u16, "Registers[5]"=→"R105":u16, "Registers[6]"=→"R106":u16, "Registers[7]"=→"R107":u16, "Registers[8]"=→"R108":u16, "Registers[9]"=→"R109":u16, "Registers[10]"=w280:u16)  [unwired: 9 out]
            n161 = local write "潜水泵工作模式"(w280) -> ()
          }
          frame "多个写入" {
            n162 = Unbundle By Name(w304) -> ("数据"=w303:variant)
            n163 = Variant To Data(type=T16 {"starting address"=0, "holding register values"=[]}, Variant=w303) -> (data=w301:T16)  [unwired: 1 in, 1 out]
            n164 = Unbundle By Name(w301) -> ("starting address"=w300:u16, "holding register values"=w299:u16[])
            n165 = call <vilib>:"Write Multiple Registers.vi"("error in (no error)"=w307, "values"=w299, "starting address"=w300, "MB session in"=w308) -> ("error out"=w306:errorcluster, "MB session out"=w305:refnum<class "MB_Master.lvclass">)  [unwired: 6 in]
          }
          frame "单个写入" {
            n166 = Unbundle By Name(w314) -> ("数据"=w313:variant)
            n167 = Variant To Data(type=T17 {"starting address"=0, "holding register value"=0}, Variant=w313) -> (data=w311:T17)  [unwired: 1 in, 1 out]
            n168 = Unbundle By Name(w311) -> ("starting address"=w310:u16, "holding register value"=w309:u16)
            n169 = call <vilib>:"Write Single Register.vi"("error in (no error)"=w317, "value"=w309, "address"=w310, "MB session in"=w318) -> ("error out"=w316:errorcluster, "MB session out"=w315:refnum<class "MB_Master.lvclass">)  [unwired: 6 in]
          }
          frame "线圈写入" {
            n170 = Unbundle By Name(w324) -> ("数据"=w323:variant)
            n171 = Variant To Data(type=T18 {"starting address"=0, "coil values"=[]}, Variant=w323) -> (data=w321:T18)  [unwired: 1 in, 1 out]
            n172 = Unbundle By Name(w321) -> ("starting address"=w320:u16, "coil values"=w319:bool[])
            n173 = call <vilib>:"Write Multiple Coils.vi"("error in (no error)"=w327, "values"=w319, "starting address"=w320, "MB session in"=w328) -> ("error out"=w326:errorcluster, "MB session out"=w325:refnum<class "MB_Master.lvclass">)  [unwired: 6 in]
          }
          frame "shutdown" {
          }
        }
      }
      frame Error {
        n174 = Unbundle By Name(w336) -> ("code"=w338:i32)
        n175 = case shown="-1073807343" w338 {
          tunnel: w337 -> [w340 w344]
          tunnel: w336 -> [w339 w346]
          tunnel: [w339 w345] -> w334
          tunnel: [w340 w344] -> w335
          tunnel: w332 -> [_ w343]
          frame Default {
          }
          frame -1073807343 {
            n176 = Flush Queue(queue=w343) -> (queue out=w342:refnum<queue>)  [unwired: 1 in, 2 out]
            n177 = call-dynamic "Close Session.vi"("error in (no error)"=w346, "MB session in"=w344) -> ("error out"=w345:errorcluster)  [unwired: 9 in]
            n178 = disable-structure shown="禁用" {
              disable-tunnel: w342 -> [w347 _]
              frame Disabled {
                n179 = Enqueue Element At Opposite End(queue=w347, element=cluster{"命令":string, "数据":variant} {"命令"="init", "数据"=variant} ("元素")) -> ()  [unwired: 2 in, 3 out]
              }
              frame Enabled {
              }
            }
            n180 = Wait (ms)(milliseconds to wait=u32 2000 ("等待时间（毫秒）")) -> ()  [unwired: 1 out]
          }
        }
        n181 = call <vilib>:"Clear Errors.vi"("error in (no error)"=w334) -> ("error out"=w333:errorcluster)  [unwired: 5 in, 1 out]
      }
    }
  }
  n182 = property on="多列列表框" class="MCListbox (严格)"("ItemNames"=string[][] [["待机"], ["初始化"], ["外部管路润洗"], ["内部管路润洗"], ["采样"], ["沉淀"], ["配水"], ["外部管路反冲洗"], ["内部管路反冲洗"], ["采样池储水"], ["结束"]] ("项名")) -> ()  [unwired: 2 in, 2 out]
  n183 = call-dynamic "Close Session.vi"("error in (no error)"=w2, "MB session in"=w1) -> ()  [unwired: 9 in, 1 out]
